vi "More Rabi.vi"() -> ()   [LabVIEW 2020]
uses:
  Labview Library/Libraries/PIScanner_new/Library/PIScanner.lvlib
  Labview Library/Libraries/Basic Experiment/Basic Experiment.lvlib
  Labview Library/Libraries/Save Module/Libraries/Save Module/Save Module.lvlib
  Labview Library/Libraries/Basic Experiment/Rabi Settings.ctl
panel:
  in  "Rabi setting section":T1={"freq(MHz)"=1378.0, "Num Pts"=60, "dBm"=-27.0, "tau start"=0.0, "tau end"=2e-06, "Loop Time"=1000, "Loop per Update"=1000} {"Loop per Update" format="%.0p"; "Loop Time" format="%.0p"; "tau end" format="%#_6p"}
  in  "Array":T2(array[cluster])=[{"Position"=[163.75, 50.4], "Freq(MHz)"=1335.0, "Count"=0.0}, {"Position"=[163.9, 41.1], "Freq(MHz)"=1370.0, "Count"=0.0}, {"Position"=[160.25, 43.4], "Freq(MHz)"=1400.0, "Count"=0.0}, {"Position"=[149.4, 45.1], "Freq(MHz)"=1375.0, "Count"=0.0}, {"Position"=[137.4, 46.7], "Freq(MHz)"=1380.0, "Count"=70.0}, {"Position"=[105.0, 47.6], "Freq(MHz)"=1375.0, "Count"=80.0}, {"Position"=[89.2, 41.3], "Freq(MHz)"=1373.0, "Count"=70.0}, {"Position"=[37.9, 42.4], "Freq(MHz)"=1376.0, "Count"=70.0}, {"Position"=[16.8, 43.2], "Freq(MHz)"=1375.0, "Count"=65.0}]
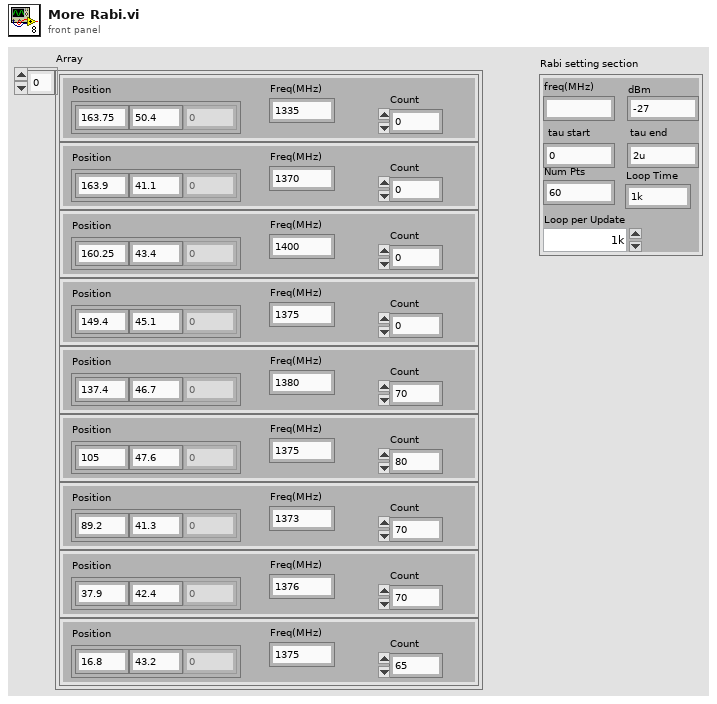
[diagram p1: front panel]
types:
  T1 = typedef "Basic Experiment.lvlib/Rabi Settings.ctl" = cluster{"freq(MHz)":ext, "Num Pts":i32, "dBm":dbl, "tau start":dbl, "tau end":dbl, "Loop Time":u32, "Loop per Update":u32}
  T2 = cluster{"Position":dbl[], "Freq(MHz)":dbl, "Count":dbl}[]
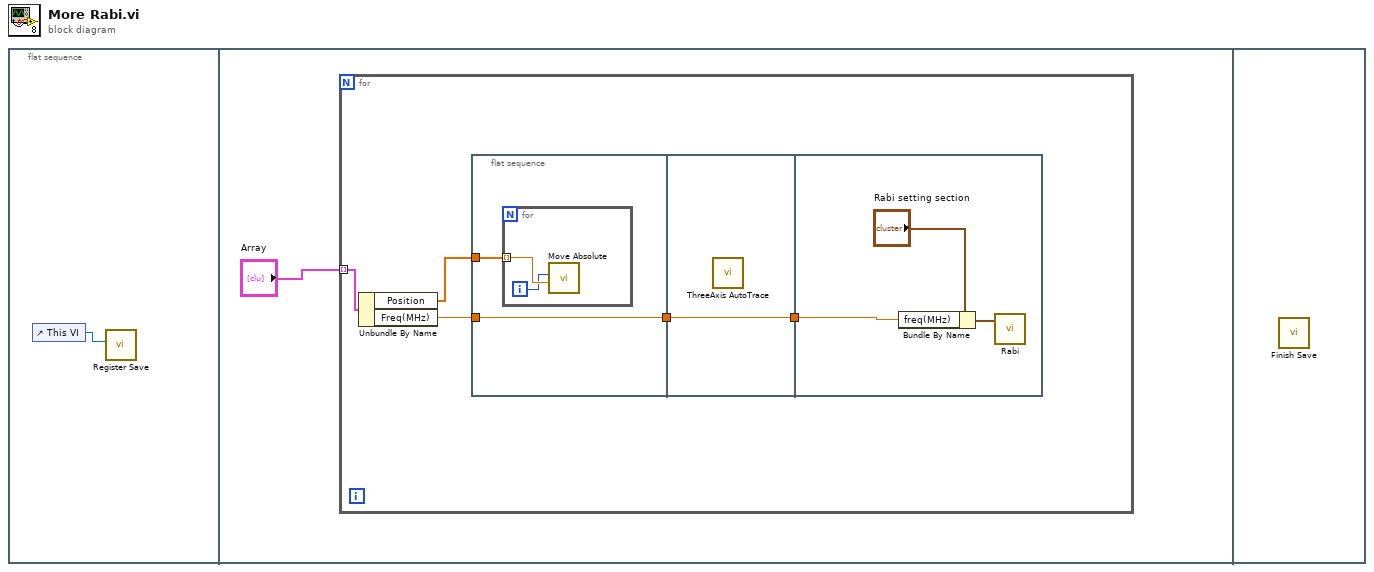
[diagram p0: block diagram]
diagram:
  n1 = flat-sequence {
    frame #0 {
      n2 = control-ref of="This VI"() -> (w1:refnum<vi>)
      n3 = call "Register Save.vi"("VI Refnum"=w1) -> ()  [unwired: 9 in, 2 out]
    }
    frame #1 {
      n4 = for {
        tunnel: "Array" -> [w7] mode=indexing
        n5 = Unbundle By Name(w7) -> ("Position"=w5:dbl[], "Freq(MHz)"=w6:dbl)
        n6 = flat-sequence {
          tunnel: w6 -> [w9]
          tunnel: [w9] -> w4
          tunnel: w5 -> [w8]
          tunnel: w4 -> [w12]
          tunnel: [w12] -> w3
          tunnel: w3 -> [w14]
          frame #0 {
            n7 = for {
              tunnel: w8 -> [w11] mode=indexing
              i -> [w10]
              n8 = call "Move Absolute.vi"("Goal Position"=w11, "Axis To Move"=w10) -> ()  [unwired: 8 in, 2 out]
            }
          }
          frame #1 {
            n9 = call "ThreeAxis AutoTrace.vi"() -> ()  [unwired: 9 in, 1 out]
          }
          frame #2 {
            n10 = Bundle By Name(cluster="Rabi setting section", "freq(MHz)"=w14) -> (w13:T1)
            n11 = call "Rabi.vi"("Rabi setting section"=w13) -> ()  [unwired: 9 in, 2 out]
          }
        }
      }
    }
    frame #2 {
      n12 = call "Finish Save.vi"() -> ()  [unwired: 11 in, 1 out]
    }
  }
